vi "Scan Setup.vi"(8 "error in (no error)":errorcluster, 11 "DAQ Digital Code Scan in":refnum<class "DAQ Digital Code Scan.lvclass">) -> (0 "error out":errorcluster, 3 "DAQ Digital Code Scan out":refnum<class "DAQ Digital Code Scan.lvclass">)   [LabVIEW 2012, in "DAQ Digital Code Scan.lvclass"]
doc: "Configure the Instrument based on the class member fields. This step comes after the user has closed the \"Scan Setup\" window and before the actual scan -- so instruments are configured with the user's specified settings."
uses:
  DAQ Digital Code Scan.lvclass
  Scanner/Scanner.lvclass
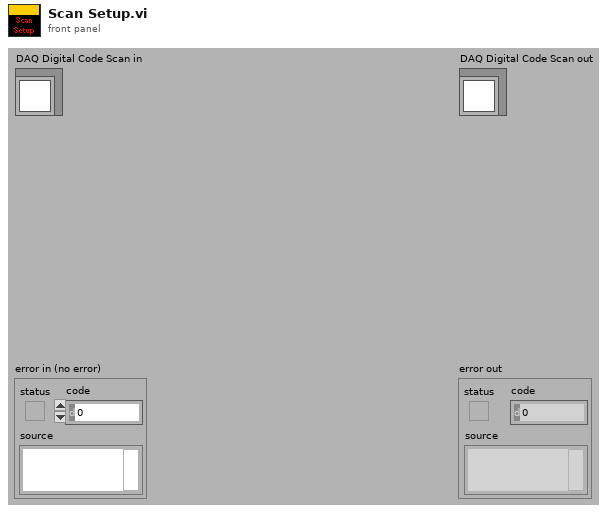
[diagram p1: front panel]
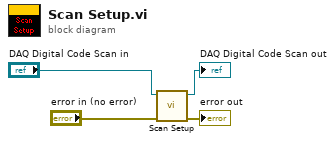
[diagram p0: block diagram]
diagram:
  n1 = call-parent "Scan Setup.vi"("error in (no error)"="error in (no error)", "Scanner in"="DAQ Digital Code Scan in") -> ("error out"=→"error out":errorcluster, "Scanner out"=→"DAQ Digital Code Scan out":refnum<class "DAQ Digital Code Scan.lvclass">)  [unwired: 8 in]
